vi "Create Header and Table Definition Constant.vi"(8 "Error In":errorcluster, 11 "Header Cluster":T1) -> (0 "Error Out":errorcluster, 3 "Output Header and Table Constant":string)   [LabVIEW 2017]
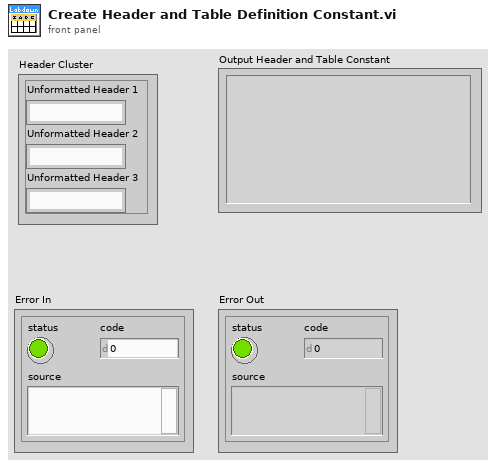
[diagram p1: front panel]
types:
  T1 = cluster{"Unformatted Header 1":string, "Unformatted Header 2":string, "Unformatted Header 3":string}
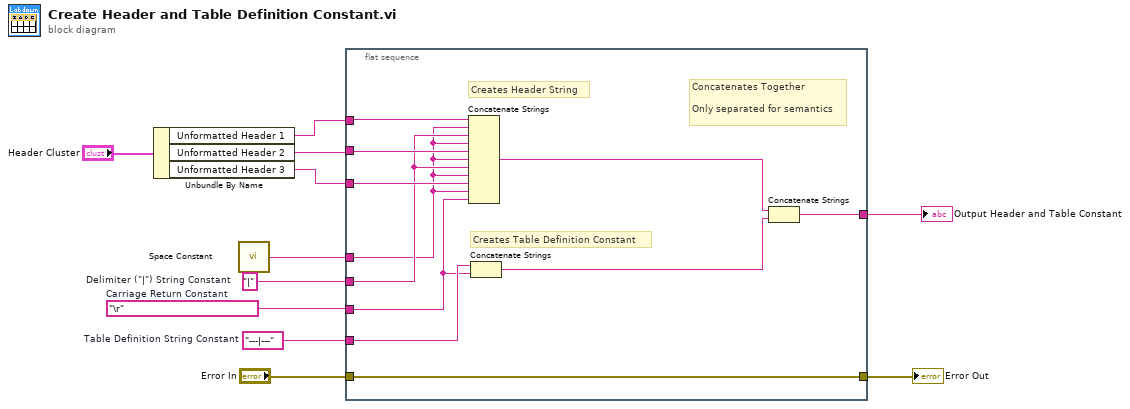
[diagram p0: block diagram]
diagram:
  w9 = "---|---"  # Table Definition String Constant
  w8 = "\r"  # Carriage Return Constant
  w11 = "|"  # Delimiter ("|") String Constant
  n1 = Unbundle By Name("Header Cluster") -> ("Unformatted Header 1"=w3:string, "Unformatted Header 2"=w2:string, "Unformatted Header 3"=w1:string)
  n2 = call <vilib>:"Space Constant.vi"() -> ("String"=w10:string)
  n3 = flat-sequence {
    tunnel: w3 -> [w22]
    tunnel: w2 -> [w21]
    tunnel: w1 -> [w20]
    tunnel: w11 -> [w19]
    tunnel: w10 -> [w18]
    tunnel: w9 -> [w17]
    tunnel: w8 -> [w12]
    tunnel: "Error In" -> [w16]
    tunnel: [w16] -> w6
    tunnel: [w13] -> w5
    frame #0 {
      # "Concatenates Together\n\nOnly separated for semantics"
      # "Creates Table Definition Constant"
      # "Creates Header String"
      n4 = Concatenate Strings(w22, w18, w19, w18, w21, w18, w19, w18, w20, w18, w12) -> (w15:string)
      n5 = Concatenate Strings(w17, w12) -> (w14:string)
      n6 = Concatenate Strings(w15, w14) -> (w13:string)
    }
  }
  "Error Out" <- w6
  "Output Header and Table Constant" <- w5
